vi "Gear Controller.vi"(8 "error in":errorcluster) -> ()   [LabVIEW 2015]
doc: "This VI executes continuously carrying out the current operation and responding to updates or new operations. It will often contain the timing or control code that is difficult to place directly in TeleOp. This VI generally opens all sensors and motors and isolates the rest of the robot code from knowing how the operations are carried out."
uses:
  Gear.ctl
  Gear Setpoints.ctl
  Gear Operations.ctl
  <vilib>/Rock Robotics/WPI/Solenoid/WPI_SolenoidChannel.ctl
  <vilib>/Rock Robotics/WPI/Solenoid/WPI_SolenoidValue.ctl
  <vilib>/Rock Robotics/WPI/Solenoid/WPI_SolenoidOpenSingle.vi
  <vilib>/Rock Robotics/WPI/Solenoid/WPI_SolenoidSetEnum.vi
  <vilib>/Rock Robotics/Network Tables/NT Write Boolean.vi
panel:
  out "Gear":T1
  out "Current\nCmd":string
  # "Tip: It may be helpful to observe inputs and sensor values.\nYou may also want to display tuning or debugging controls."
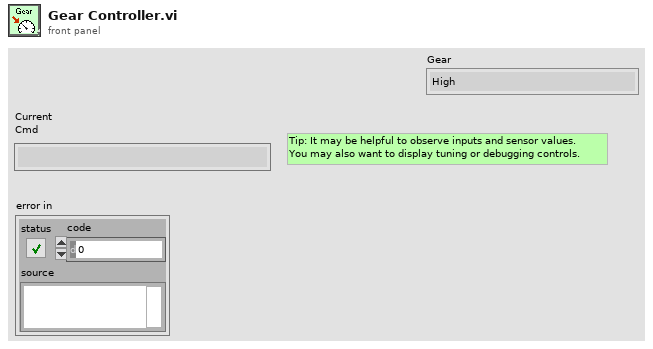
[diagram p1: front panel]
types:
  T1 = typedef "Gear.ctl" = enum16{"High", "Low"}
  T2 = typedef "WPI_SolenoidChannel.ctl" = enum8{"Solenoid 0", "Solenoid 1", "Solenoid 2", "Solenoid 3", "Solenoid 4", "Solenoid 5", "Solenoid 6", "Solenoid 7", "Invalid"}
  T3 = typedef "Gear Setpoints.ctl" = cluster{"Operation":T4, "Setpoint":dbl, "Duration":dbl, "Gear":T1}
  T4 = typedef "Gear Operations.ctl" = enum16{"Reserve", "Read Current", "Immediate", "Change Gear"}
  T5 = typedef "WPI_CompressorDevRef.ctl" = cluster{"DevStatus":errorcluster, "Pneumatics Control Module":u8}
  T6 = typedef "WPI_SolenoidDevRef.ctl" = cluster{"DevStatus":errorcluster, "Pneumatics Control Module":u8, "Forward Solenoid Channel":T2, "Reverse Solenoid Channel":T2}
  T7 = typedef "Command Status Info.ctl" = cluster{"Name":string, "Status":T8, "notifier out":T9}
  T8 = typedef "Completion Status.ctl" = enum16{"Successful", "Aborted", "Incomplete"}
  T9 = typedef "Completion Notifier.ctl" = refnum<notifier>
  T10 = cluster{"Default Command":T3, "Command Timing":cluster{"Start Time (ms)":u32, "Iterations":i32}, "Command Arguments":cluster{"Command Info":T7, "Description":string, "Default Command":T3, "notifier out":refnum<notifier>, "Subsystem Name":string}}
  T11 = typedef "WPI_SolenoidValue.ctl" = enum16{"Off", "On", "Forward", "Reverse"}
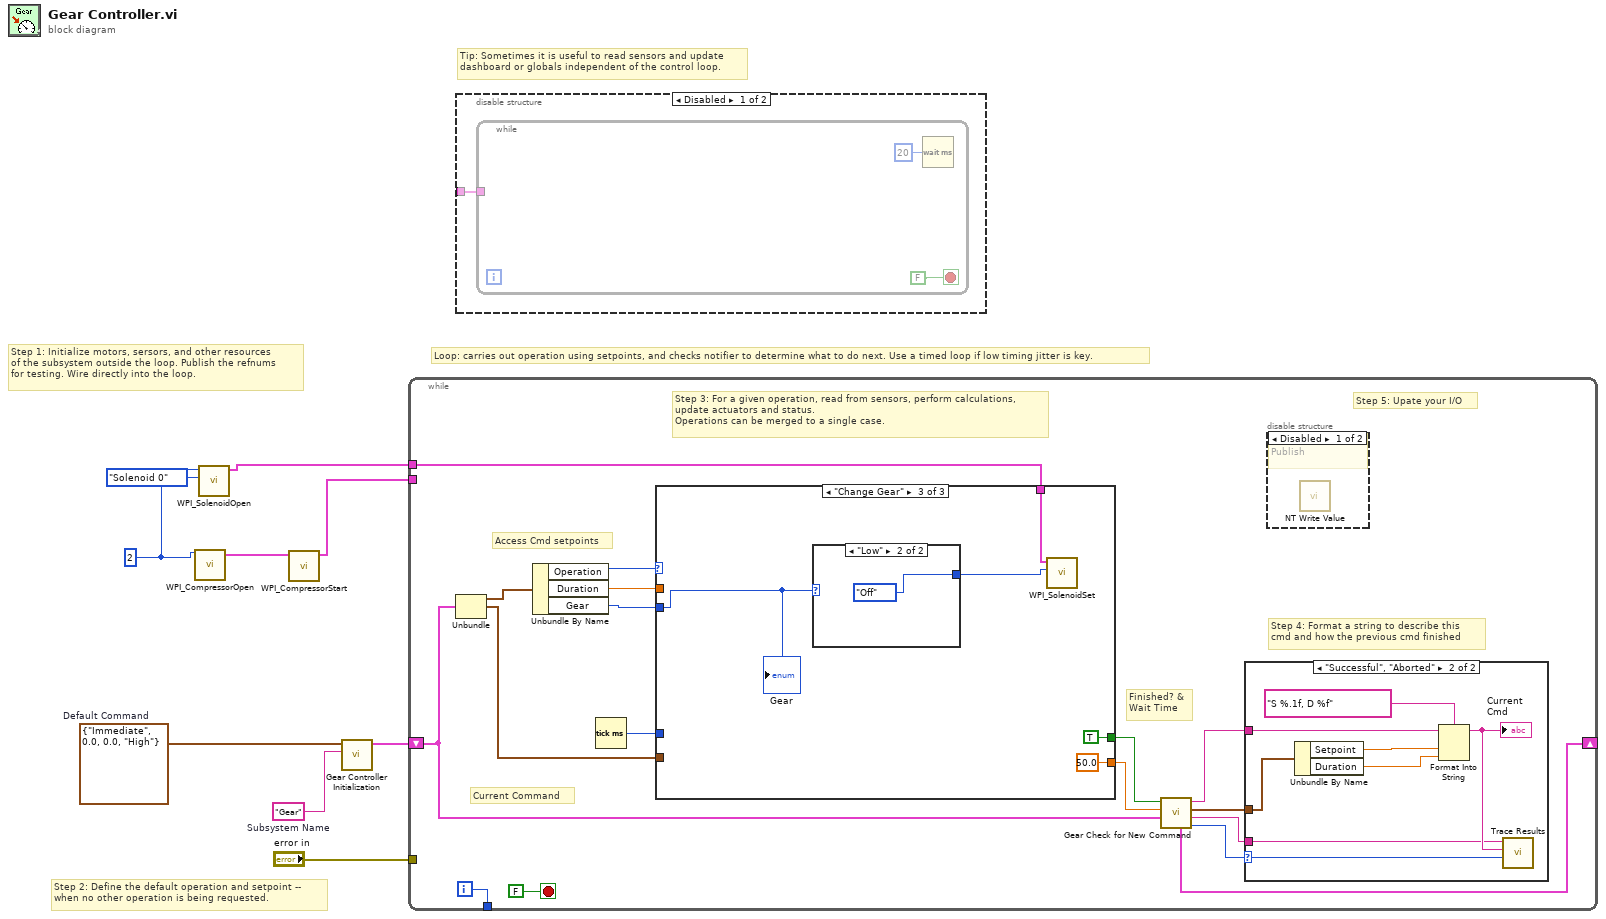
[diagram p0: block diagram]
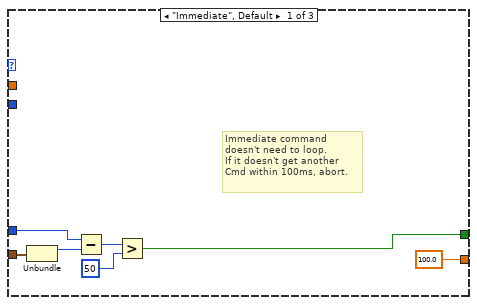
[diagram p5: hidden frame]
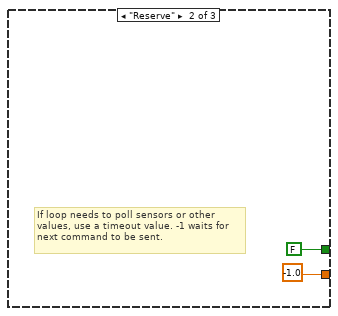
[diagram p6: hidden frame]
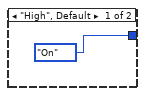
[diagram p7: hidden frame]
diagram:
  w3 = u8 2 ("Pneumatics Control Module (0)")
  w6 = T3 {"Operation"=enum."Immediate", "Setpoint"=0.0, "Duration"=0.0, "Gear"=enum."High"}  # Default Command
  w7 = "Gear"  # Subsystem Name
  # "Tip: Sometimes it is useful to read sensors and update\ndashboard or globals independent of the control loop."
  # "Step 2: Define the default operation and setpoint --\nwhen no other operation is being requested."
  # "Step 1: Initialize motors, sersors, and other resources\nof the subsystem outside the loop. Publish the refnums\nfor testing. Wire directly into the loop."
  # "Loop: carries out operation using setpoints, and checks notifier to determine what to do next. Use a timed loop if low timing jitter is key."
  n1 = call <vilib>:"WPI_CompressorOpen.vi"("Pneumatics Control Module (0)"=w3) -> ("CompressorDevRef"=w5:T5)  [unwired: 13 in, 1 out]
  n2 = call-poly <vilib>:"WPI_SolenoidOpen.vi"("Solenoid Channel"=WPI_SolenoidChannel."Solenoid 0", "Pneumatics Control Module (0)"=w3) -> ("SolenoidDevRef"=w1:T6)  [unwired: 8 in, 1 out]
  n3 = call <vilib>:"WPI_CompressorStart.vi"("CompressorDevRef"=w5) -> ("CompressorDevRef"=w4:T5)  [unwired: 9 in, 1 out]
  n4 = call "Gear Controller Initialization.vi"("Subsystem Name"=w7, "Default Command"=w6) -> ("Command Info"=w8:T10)  [unwired: 9 in]
  n5 = while {
    shift-right: [w17] -> _
    shift-left: w8 -> [w18]
    tunnel: [w25] -> _
    tunnel: "error in" -> [_]
    tunnel: w4 -> [_]
    tunnel: w1 -> [w10]
    i -> [w25]
    stop <- FALSE stop-if-true
    # "Step 5: Upate your I/O"
    # "Step 4: Format a string to describe this\ncmd and how the previous cmd finished"
    # "Current Command"
    # "Access Cmd setpoints"
    # "Finished? &\nWait Time"
    # "Step 3: For a given operation, read from sensors, perform calculations,\nupdate actuators and status.\nOperations can be merged to a single case."
    n6 = Unbundle(w18) -> ("Default Command"=w24:T3, "Command Timing"=w20:cluster{"Start Time (ms)":u32, "Iterations":i32})  [unwired: 1 out]
    n7 = Unbundle By Name(w24) -> ("Operation"=w23:T4, "Duration"=w22:dbl, "Gear"=w19:T1)
    n8 = Tick Count (ms)() -> (millisecond timer value=w21:u32)
    n9 = case shown="\"Change Gear\"" w23 {
      tunnel: [100.0 -1.0 50.0] -> w15
      tunnel: [w35 FALSE ("ignore previous (F)") TRUE ("ignore previous (F)")] -> w16
      tunnel: w20 -> [w37 _ _]
      tunnel: w22 -> [_ _ _]
      tunnel: w21 -> [w36 _ _]
      tunnel: w19 -> [_ _ w48]
      tunnel: w10 -> [_ _ w47]
      frame "Immediate", Default {
        # "Immediate command\ndoesn't need to loop.\nIf it doesn't get another\nCmd within 100ms, abort."
        n10 = Unbundle(w37) -> ("Start Time (ms)"=w40:u32)  [unwired: 1 out]
        n11 = Subtract(x=w36, y=w40) -> (x-y=w39:u32)
        n12 = Greater?(x=w39, y=u8 50 ("Left Motor")) -> (0:w35:bool)
      }
      frame "Reserve" {
        # "If loop needs to poll sensors or other\nvalues, use a timeout value. -1 waits for\nnext command to be sent."
      }
      frame "Change Gear" {
        n13 = case shown="\"Low\"" w48 {
          tunnel: [WPI_SolenoidValue."On" ("Value") WPI_SolenoidValue."Off" ("Value")] -> w46
          frame "High", Default {
          }
          frame "Low" {
          }
        }
        n14 = call-poly <vilib>:"WPI_SolenoidSet.vi"("Value"=w46, "SolenoidDevRef"=w47) -> ()  [unwired: 8 in, 2 out]
        "Gear" <- w48
      }
    }
    n15 = call "Gear Check for New Command.vi"("Current Command"=w18, "Wait time (ms)"=w15, "Finished?"=w16) -> ("Completion"=w11:T8, "Subsystem Name"=w12:string, "Current Command"=w13:T3, "Initial Trace String"=w14:string, "NextCommand"=w17:T10)  [unwired: 4 in]
    n16 = case shown="\"Successful\", \"Aborted\"" w11 {
      selector: w11 -> [_ w34]
      tunnel: w14 -> [_ w30]
      tunnel: w13 -> [_ w31]
      tunnel: w12 -> [_ w27]
      frame "Incomplete", Default {
        # "Continuing current command"
      }
      frame "Successful", "Aborted" {
        # "Report and setup for next command"
        n17 = Unbundle By Name(w31) -> ("Setpoint"=w33:dbl, "Duration"=w28:dbl)
        n18 = Format Into String(format string="S %.1f, D %f", initial string=w30, w33, w28) -> (resulting string=w29:string)  [unwired: 1 in, 1 out]
        "Current\nCmd" <- w29
        n19 = call <vilib>:"Trace Results.vi"("Status of previous command"=w34, "Description"=w29, "Subsystem"=w27) -> ()  [unwired: 9 in]
      }
    }
    n20 = disable-structure shown="Disabled" {
      frame Disabled {
        # "Publish"
        n21 = call-poly <vilib>:"NT Write Value.vi"() -> ()  [unwired: 11 in, 1 out]
      }
      frame Enabled {
      }
    }
  }
  n22 = disable-structure shown="Disabled" {
    disable-tunnel: _ -> [w51 _]
    frame Disabled {
      n23 = while {
        tunnel: w51 -> [_]
        stop <- FALSE stop-if-true
        n24 = Wait (ms)(milliseconds to wait=u32 20) -> ()  [unwired: 1 out]
      }
    }
    frame Enabled {
    }
  }
